vi "Position Plot.vi"(10 "Force Arrow":dbl[](array[numeric]), 11 "Measured Position":dbl[](array[numeric])) -> (2 "Force Arrow":cluster{dbl[], dbl[]}, 3 "X,Y":cluster{dbl[], dbl[]})   [LabVIEW 2021]
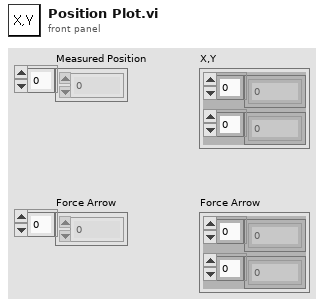
[diagram p1: front panel]
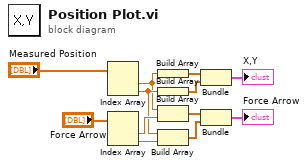
[diagram p0: block diagram]
diagram:
  n1 = Index Array(array="Measured Position") -> (element #1=w4:dbl, element #2=w5:dbl)  [unwired: 2 in]
  n2 = Index Array(array="Force Arrow") -> (element #1=w9:dbl, element #2=w10:dbl)  [unwired: 2 in]
  n3 = Build Array(w4) -> (w1:dbl[])
  n4 = Build Array(w5) -> (w2:dbl[])
  n5 = Build Array(w4, w9) -> (w6:dbl[])
  n6 = Build Array(w5, w10) -> (w7:dbl[])
  n7 = Bundle(w1, w2) -> (→"X,Y":cluster{dbl[], dbl[]})  [unwired: 1 in]
  n8 = Bundle(w6, w7) -> (→"Force Arrow":cluster{dbl[], dbl[]})  [unwired: 1 in]
